vi "GetStageMotionStatusDll.vi"(8 "error in":errorcluster, 9 "Stage":T1, 11 "DevRefIn":u32) -> (0 "error out":errorcluster, 1 "Moving":bool, 2 "Stage Position":string, 3 "DevRefOut":u32)   [LabVIEW 2020]
uses:
  StageSelector--Enum.ctl
  Galil/resources/gclib32/gclib32.lvlib
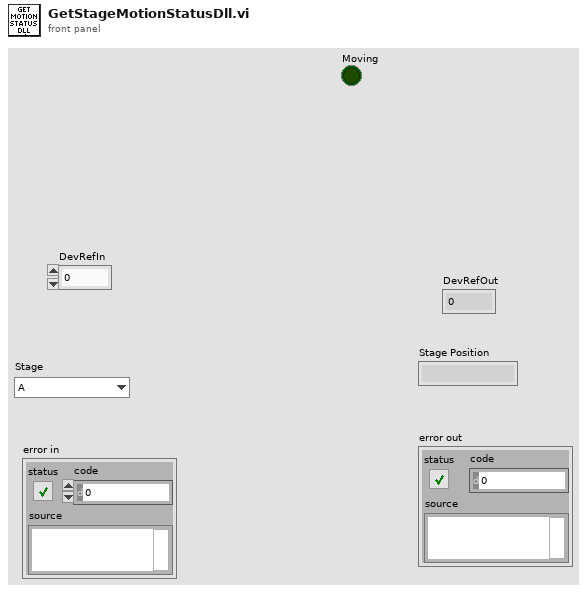
[diagram p1: front panel]
types:
  T1 = typedef "StageSelector--Enum.ctl" = enum16{"A", "B", "C", "D"}
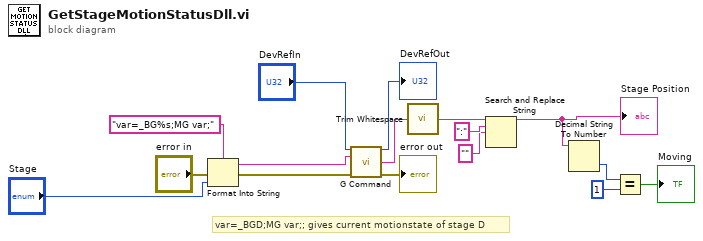
[diagram p0: block diagram]
diagram:
  # "var=_BGD;MG var;; gives current motionstate of stage D"
  n1 = Format Into String(format string="var=_BG%s;MG var;", error in="error in", "Stage") -> (resulting string=w8:string, error out=w9:errorcluster)  [unwired: 1 in]
  n2 = call "G Command.vi"("g"="DevRefIn", "command"=w8, "error in (no error)"=w9) -> ("g out"=→"DevRefOut":u32, "buffer out"=w6:string, "error out"=→"error out":errorcluster)  [unwired: 10 in]
  n3 = call <vilib>:"Trim Whitespace.vi"("string"=w6) -> ("trimmed string"=w15:string)  [unwired: 1 in]
  n4 = Search and Replace String(input string=w15, search string=":", replace string="" ("replace string (\"\")")) -> (result string=w4:string)  [unwired: 5 in, 3 out]
  "Stage Position" <- w4
  n5 = Decimal String To Number(string=w4) -> (number=w3:i32)  [unwired: 2 in, 1 out]
  n6 = Equal?(x=w3, y=1) -> (x = y?=→"Moving":bool)
